vi "rad_Load Targets from File.vi"(11 "PathFile":path) -> (1 "Valid File":bool, 3 "IPs to Load":string[](array[string]))   [LabVIEW 2016]
doc: "Opens the provided txt file and returns a list with the IP Addresses found. IPs are expected to be in the format xx.xx.xx.xx. IPs with different format will be filtered. s"
uses:
  <vilib>/Utility/file.llb/Read Delimited Spreadsheet (string).vi
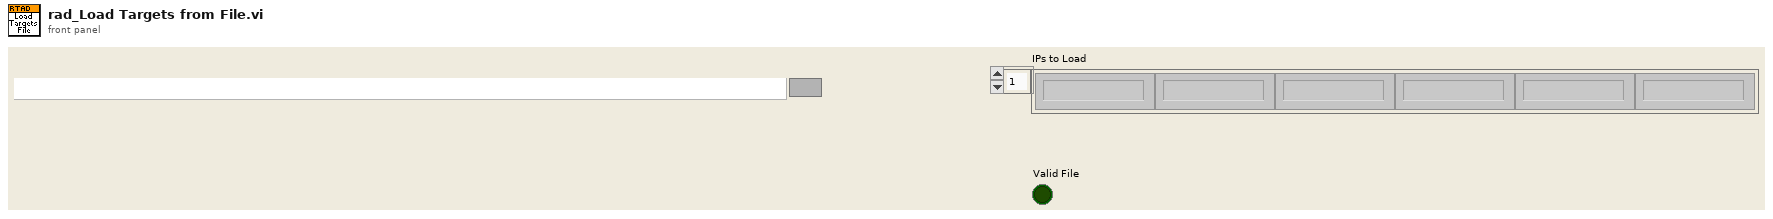
[diagram p1: front panel]
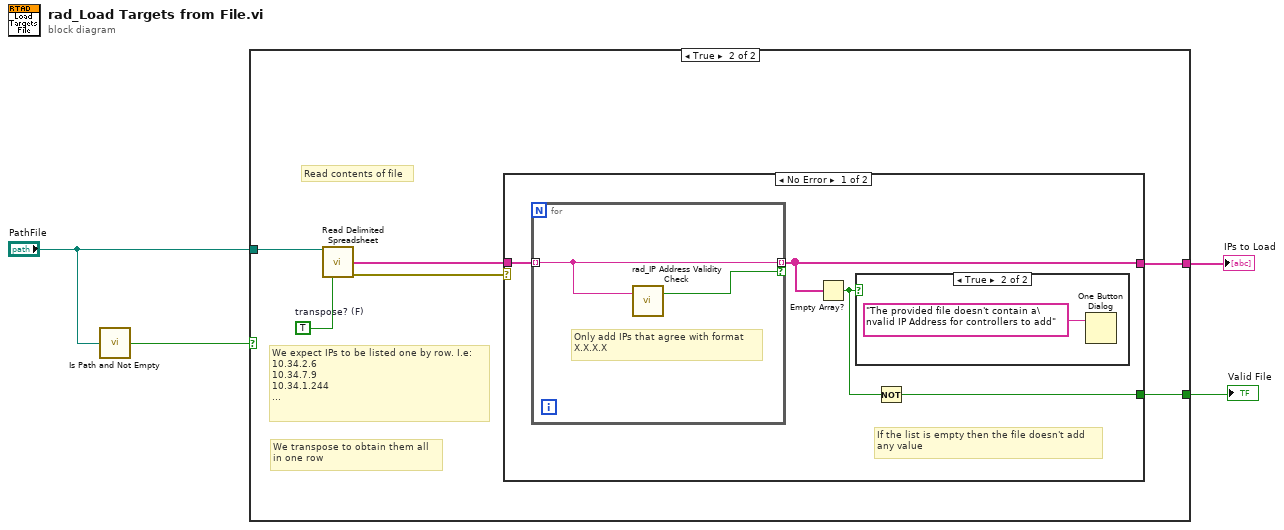
[diagram p0: block diagram]
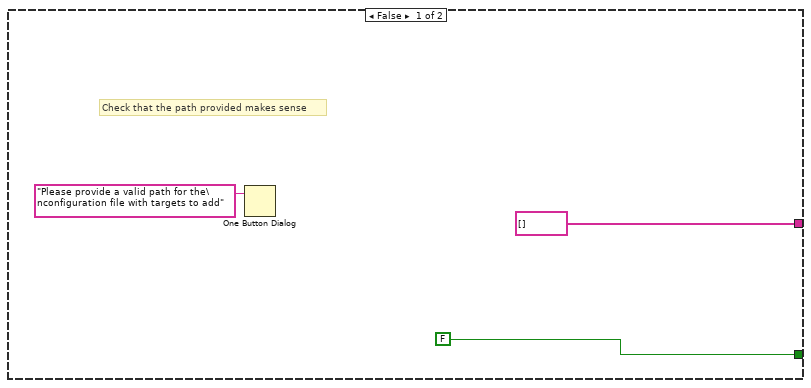
[diagram p2: hidden frame]
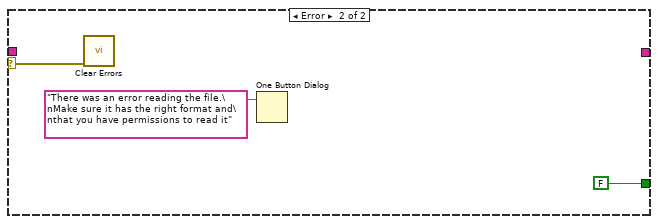
[diagram p4: hidden frame]
diagram:
  n1 = call <vilib>:"Is Path and Not Empty.vi"("path"="PathFile") -> ("Is Path and Not Empty?"=w3:bool)  [unwired: 4 in]
  n2 = case shown="True" w3 {
    tunnel: "PathFile" -> [_ w13]
    tunnel: [FALSE w10] -> w2
    tunnel: [string[] [] w8] -> w1
    frame False {
      # "Check that the path provided makes sense"
      n3 = One Button Dialog(message="Please provide a valid path for the\nconfiguration file with targets to add") -> ()  [unwired: 1 in, 1 out]
    }
    frame True {
      w11 = TRUE  # transpose? (F)
      # "We transpose to obtain them all\nin one row"
      # "We expect IPs to be listed one by row. I.e:\n10.34.2.6\n10.34.7.9\n10.34.1.244\n..."
      # "Read contents of file"
      n4 = call-poly <vilib>:"Read Delimited Spreadsheet.vi"("file path (dialog if empty)"=w13, "transpose? (F)"=w11) -> ("first row"=w9:string[], "error out"=w12:errorcluster)  [unwired: 8 in, 4 out]
      n5 = case shown="No Error" w12 {
        selector: w12 -> [_ w22]
        tunnel: [w14 FALSE] -> w10
        tunnel: w9 -> [w17 _]
        tunnel: [w16 _] -> w8
        frame No Error {
          # "If the list is empty then the file doesn't add\nany value"
          n6 = for {
            tunnel: w17 -> [w20] mode=indexing
            tunnel: [w20] -> w16 mode=indexing if=w19
            # "Only add IPs that agree with format\nX.X.X.X"
            n7 = call "rad_IP Address Validity Check.vi"("IP Address"=w20) -> ("Valid IP"=w19:bool)  [unwired: 2 in]
          }
          n8 = Empty Array?(array=w16) -> (empty?=w15:bool)
          n9 = case shown="True" w15 {
            frame False {
            }
            frame True {
              n10 = One Button Dialog(message="The provided file doesn't contain a\nvalid IP Address for controllers to add") -> ()  [unwired: 1 in, 1 out]
            }
          }
          n11 = Not(x=w15) -> (.not. x?=w14:bool)
        }
        frame Error {
          n12 = call <vilib>:"Clear Errors.vi"("error in (no error)"=w22) -> ()  [unwired: 5 in, 2 out]
          n13 = One Button Dialog(message="There was an error reading the file.\nMake sure it has the right format and\nthat you have permissions to read it") -> ()  [unwired: 1 in, 1 out]
        }
      }
    }
  }
  "IPs to Load" <- w1
  "Valid File" <- w2
